vi "Configure Integration.vi"(8 "error in (no error)":errorcluster, 10 "Integration Time (0 PLCs)":dbl, 11 "VISA resource name":refnum<visa-resource-name>) -> (0 "error out":errorcluster, 3 "VISA resource name out":refnum<visa-resource-name>)   [LabVIEW 2010, in "Agilent 3458.lvlib"]
doc: "Configures the integration time of the DMM by setting the number of PLCs (Power Line Cycles). The lesser the intergration time, the faster the measurement acquistion will be. \n\n<b>Note:</b> Setting the number of PLCs to 0 when measuring values below 1 Volt when autoranging is enabled will cause the instrument to return incorrect values when the resolution is higher than 4.5 digits. If 8.5 digits of resolution are desired, the NPLCs must be 10 or greater."
uses:
  <instrlib>/Agilent 3458/Agilent 3458.lvlib
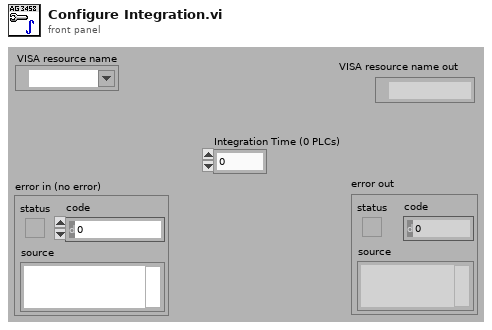
[diagram p1: front panel]
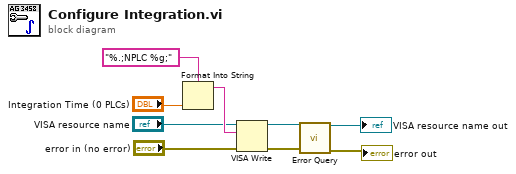
[diagram p0: block diagram]
diagram:
  n1 = Format Into String(format string="%.;NPLC %g;", "Integration Time (0 PLCs)") -> (resulting string=w6:string)  [unwired: 2 in, 1 out]
  n2 = VISA Write(VISA resource name="VISA resource name", write buffer=w6, error in (no error)="error in (no error)") -> (VISA resource name out=w8:refnum<visa-resource-name>, error out=w7:errorcluster)  [unwired: 1 out]
  n3 = call <instrlib>:"Error Query.vi"("error in (no error)"=w7, "VISA resource name"=w8) -> ("error out"=→"error out":errorcluster, "VISA resource name out"=→"VISA resource name out":refnum<visa-resource-name>)  [unwired: 6 in, 2 out]
